vi "CMD_PLACEPART.vi"(6 "Gantry in":refnum<class "Gantry.lvclass">, 8 "error in (no error)":errorcluster, 10 "Arguments":string[](array[string]), 11 "gScript Interpreter in":refnum<class "gScript Interpreter.lvclass">) -> (0 "error out":errorcluster, 3 "gScript Interpreter out":refnum<class "gScript Interpreter.lvclass">, 4 "Gantry out":refnum<class "Gantry.lvclass">)   [LabVIEW 2022 SP3, in "gScript Interpreter.lvclass"]
uses:
  gScript Interpreter.lvclass
  Shared Components/Gantry Class/Gantry.lvclass
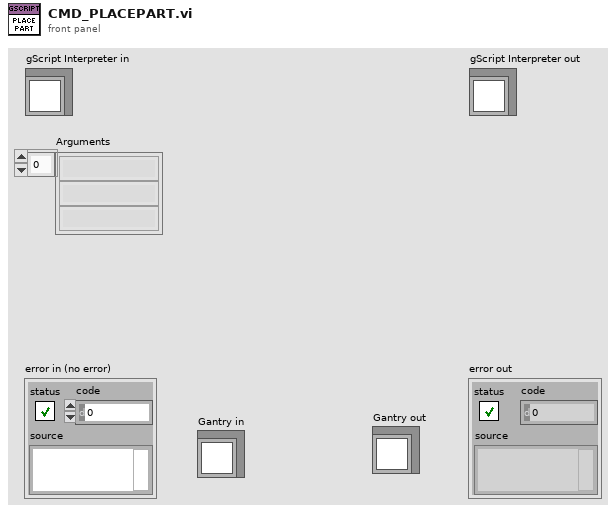
[diagram p1: front panel]
types:
  T1 = typedef "Memory Cell.ctl" = cluster{"type":T2, "x":dbl, "y":dbl, "z":dbl, "w":dbl}
  T2 = typedef "Memory Cell Type Enum.ctl" = enum16{"integer", "float", "vector", "rotation"}
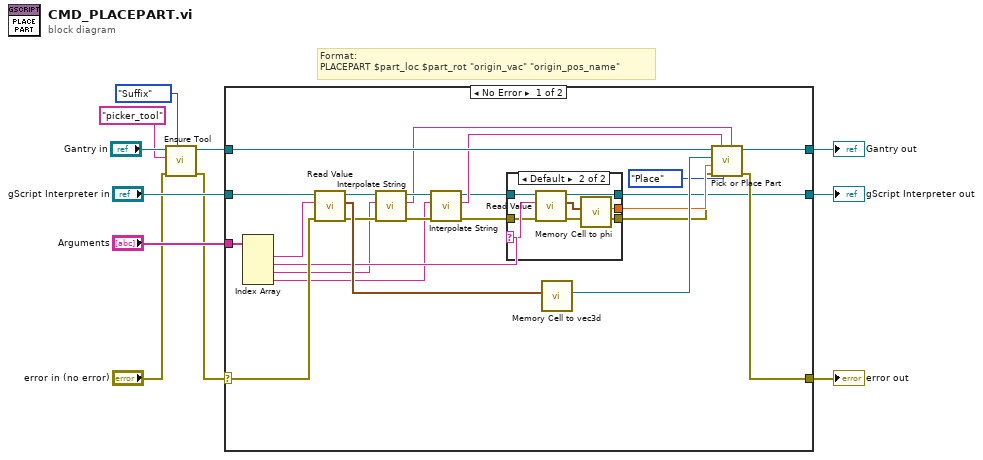
[diagram p0: block diagram]
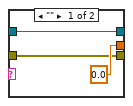
[diagram p2: hidden frame]
diagram:
  # "Format:\nPLACEPART $part_loc $part_rot \"origin_vac\" \"origin_pos_name\""
  n1 = call "Ensure Tool.vi"("Match Type"=enum16{"Full", "Suffix"}."Suffix", "error in (no error)"="error in (no error)", "Tool Name"="picker_tool", "Gantry in"="Gantry in") -> ("error out"=w3:errorcluster, "Gantry out"=w5:refnum<class "Gantry.lvclass">)  [unwired: 6 in]
  n2 = case shown="No Error" w3 {
    selector: w3 -> [w32 w48]
    tunnel: [w23 w48] -> w11
    tunnel: [w22 w47] -> w9
    tunnel: "gScript Interpreter in" -> [w34 w47]
    tunnel: "Arguments" -> [w33 _]
    tunnel: w5 -> [w29 w46]
    tunnel: [w24 w46] -> w7
    frame No Error {
      n3 = Index Array(array=w33) -> (element #1=w35:string, element #2=w30:string, element #3=w17:string, element #4=w15:string)  [unwired: 4 in]
      n4 = call-dynamic "Read Value.vi"("error in (no error)"=w32, "String in"=w35, "gScript Interpreter in"=w34) -> ("error out"=w18:errorcluster, "Memory Cell"=w31:T1, "gScript Interpreter out"=w19:refnum<class "gScript Interpreter.lvclass">)  [unwired: 6 in]
      n5 = call-dynamic "Interpolate String.vi"("error in (no error)"=w18, "Input String"=w17, "gScript Interpreter in"=w19) -> ("error out"=w20:errorcluster, "Output String"=w16:string, "gScript Interpreter out"=w21:refnum<class "gScript Interpreter.lvclass">)  [unwired: 6 in]
      n6 = call-dynamic "Interpolate String.vi"("error in (no error)"=w20, "Input String"=w15, "gScript Interpreter in"=w21) -> ("error out"=w13:errorcluster, "Output String"=w14:string, "gScript Interpreter out"=w12:refnum<class "gScript Interpreter.lvclass">)  [unwired: 6 in]
      n7 = case shown="Default" w30 {
        selector: w30 -> [_ w43]
        tunnel: w12 -> [w38 w45]
        tunnel: [w36 w44] -> w25
        tunnel: [0.0 ("float out") w41] -> w27
        tunnel: [w38 w40] -> w22
        tunnel: w13 -> [w36 w39]
        frame "" {
        }
        frame Default {
          n8 = call-dynamic "Read Value.vi"("error in (no error)"=w39, "String in"=w43, "gScript Interpreter in"=w45) -> ("error out"=w44:errorcluster, "Memory Cell"=w42:T1, "gScript Interpreter out"=w40:refnum<class "gScript Interpreter.lvclass">)  [unwired: 6 in]
          n9 = call "Memory Cell to phi.vi"("Memory Cell"=w42) -> ("float out"=w41:dbl)  [unwired: 10 in]
        }
      }
      n10 = call "Memory Cell to vec3d.vi"("Memory Cell"=w31) -> ("Vec3d out"=w28:refnum<class "Vec3d.lvclass">)  [unwired: 10 in]
      n11 = call "Pick or Place Part.vi"("Part Vacuum Line"=w16, "Pick or Place"=enum16{"Pick", "Place"}."Place", "Part Named Position"=w14, "error in (no error)"=w25, "Part Rotation"=w27, "Part Position"=w28, "Gantry in"=w29) -> ("error out"=w23:errorcluster, "Gantry out"=w24:refnum<class "Gantry.lvclass">)  [unwired: 3 in]
    }
    frame Error {
    }
  }
  "error out" <- w11
  "gScript Interpreter out" <- w9
  "Gantry out" <- w7
